vi "HardwareQueueCluster.vi"() -> ()   [LabVIEW 2017]
uses:
  HardwareQueueCluster.ctl
  hardwareMessage.ctl
panel:
  in  "HardwareQueueCluster":T1
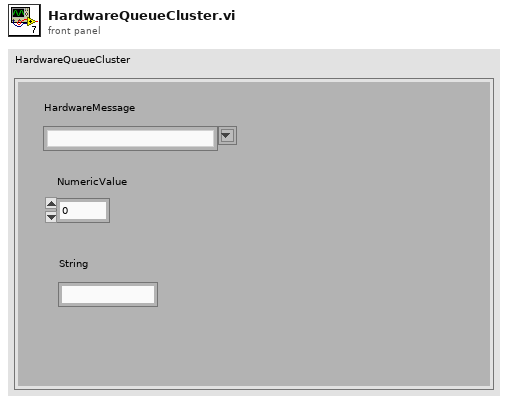
[diagram p1: front panel]
types:
  T1 = typedef "HardwareQueueCluster.ctl" = cluster{"HardwareMessage":T2, "NumericValue":dbl, "String":string}
  T2 = typedef "hardwareMessage.ctl" = string
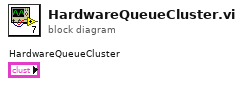
[diagram p0: block diagram]
diagram:
